vi "DOE Dryer RMC Calculation Equation.vi"(7 "Use Runtime RMC Calculation?":bool, 8 "Error In":errorcluster, 9 "Bone Dry Weight of Cloth (lbs)":dbl, 10 "Dryer Weight (lbs)":dbl, 11 "Gross Weigth (lbs)":dbl) -> (0 "Error Out":errorcluster, 1 "Relative Moisture Content-Avg (%)":dbl, 2 "Relative Moisture Content (%)":dbl, 3 "WeightCloth":dbl)   [LabVIEW 2016]
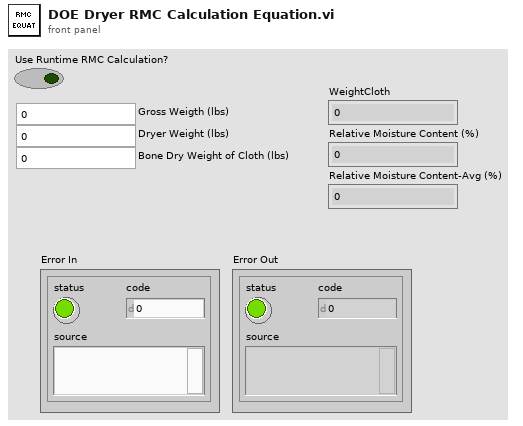
[diagram p1: front panel]
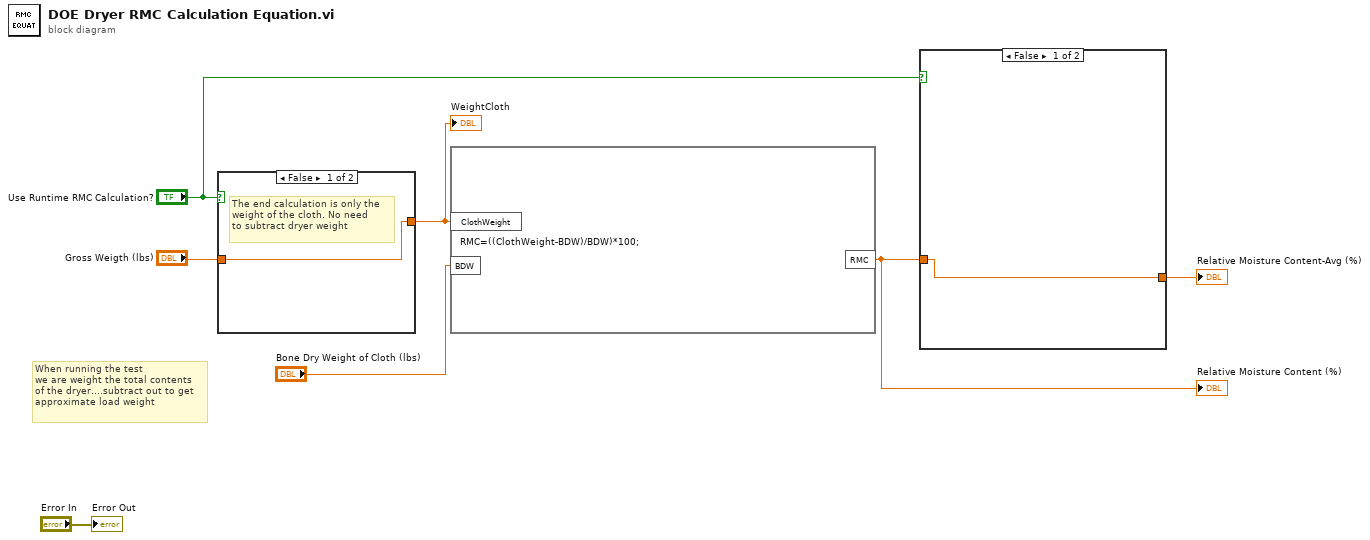
[diagram p0: block diagram]
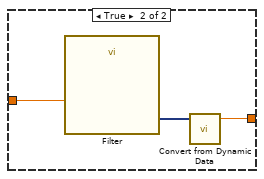
[diagram p2: hidden frame]
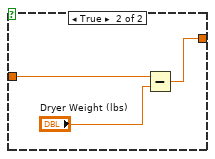
[diagram p3: hidden frame]
diagram:
  # "When running the test\nwe are weight the total contents\nof the dryer....subtract out to get\napproximate load weight"
  n1 = case shown="False" "Use Runtime RMC Calculation?" {
    tunnel: [w8 w10] -> w5
    tunnel: "Gross Weigth (lbs)" -> [w8 w9]
    frame False {
      # "The end calculation is only the\nweight of the cloth. No need\nto subtract dryer weight"
    }
    frame True {
      n2 = Subtract(x=w9, y="Dryer Weight (lbs)") -> (x-y=w10:dbl)
    }
  }
  "WeightCloth" <- w5
  n3 = formula code="RMC=((ClothWeight-BDW)/BDW)*100;"("BDW"="Bone Dry Weight of Cloth (lbs)", "ClothWeight"=w5) -> ("RMC"=w4:dbl)
  "Relative Moisture Content (%)" <- w4
  n4 = case shown="False" "Use Runtime RMC Calculation?" {
    tunnel: w4 -> [w12 w14]
    tunnel: [w12 w13] -> w3
    frame False {
    }
    frame True {
      n5 = call "Filter"("Signal"=w14) -> ("Filtered Signal"=w15:dynamicdata)  [unwired: 9 in, 1 out]
      n6 = call "Convert from Dynamic Data"("Dynamic Data Type"=w15) -> ("Scalar"=w13:dbl)  [unwired: 3 in]
    }
  }
  "Relative Moisture Content-Avg (%)" <- w3
  "Error Out" <- "Error In"
